vi "QModbus.vi"(9 "Main Process Class in":refnum<class "Main Class.lvclass">) -> ()   [LabVIEW 2019]
uses:
  Main Class.lvclass
  LLB/Commonly VI/Main Glb.vi
  LLB/Commonly VI.lvlib
  Ctrl/ModbusCmd.ctl
  <vilib>/NI/Modbus Library/API/Master/Modbus Master.lvclass
panel:
  out "error IO":errorcluster
  in  "Boolean":bool
  out "Main Process Class out":refnum<class "Main Class.lvclass">
  out "queue out":refnum<queue>
  out "register values":u16[](array[numeric])
  out "discrete inputs":bool[](array[boolean])
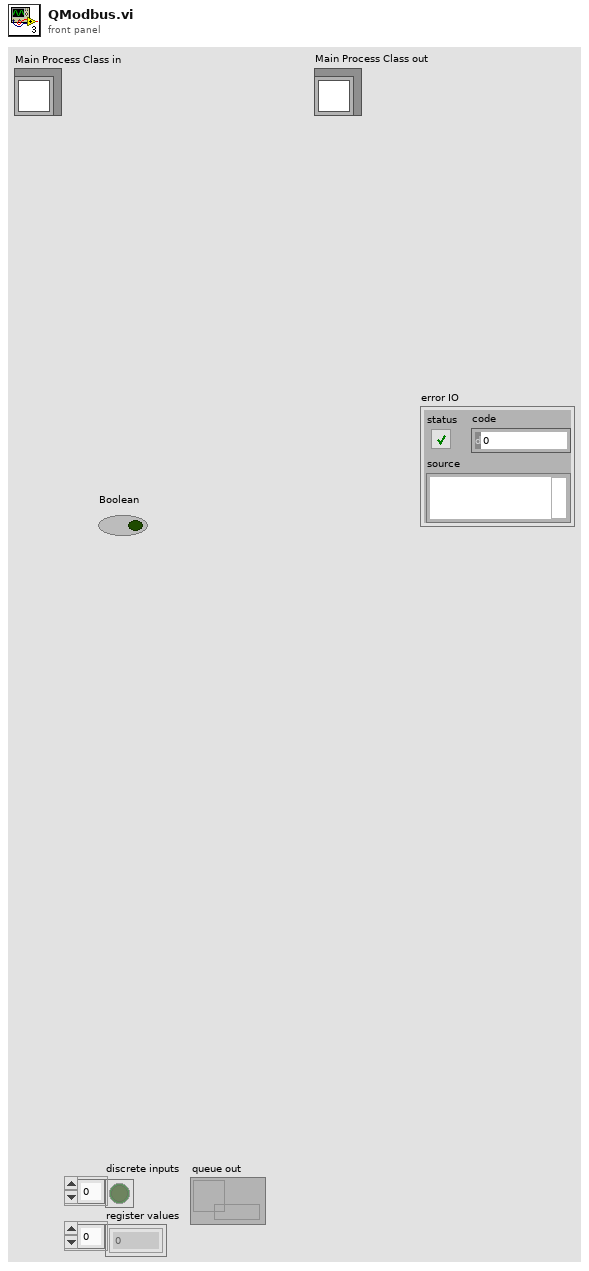
[diagram p1: front panel]
types:
  T1 = cluster{"AutoRunFlg":refnum<vi>, "Action Finish Flg":refnum<vi>, "Remaining Action":refnum<vi>, "Btn_AutoRun":refnum<vi>, "Manual Flg":refnum<vi>, "Sub Process Error":refnum<vi>}
  T2 = cluster{"starting address":u16, "coils to write":bool[]}
  T3 = typedef "ModbusCmd.ctl" = enum16{"Connect", "Disconnect", "Init", "Fetch Basic Objects", "Fetch Input Refisters", "Fetch Discrete Inputs", "Set Coils", "Set Holding Registers", "Write Single Holding", "Exit"}
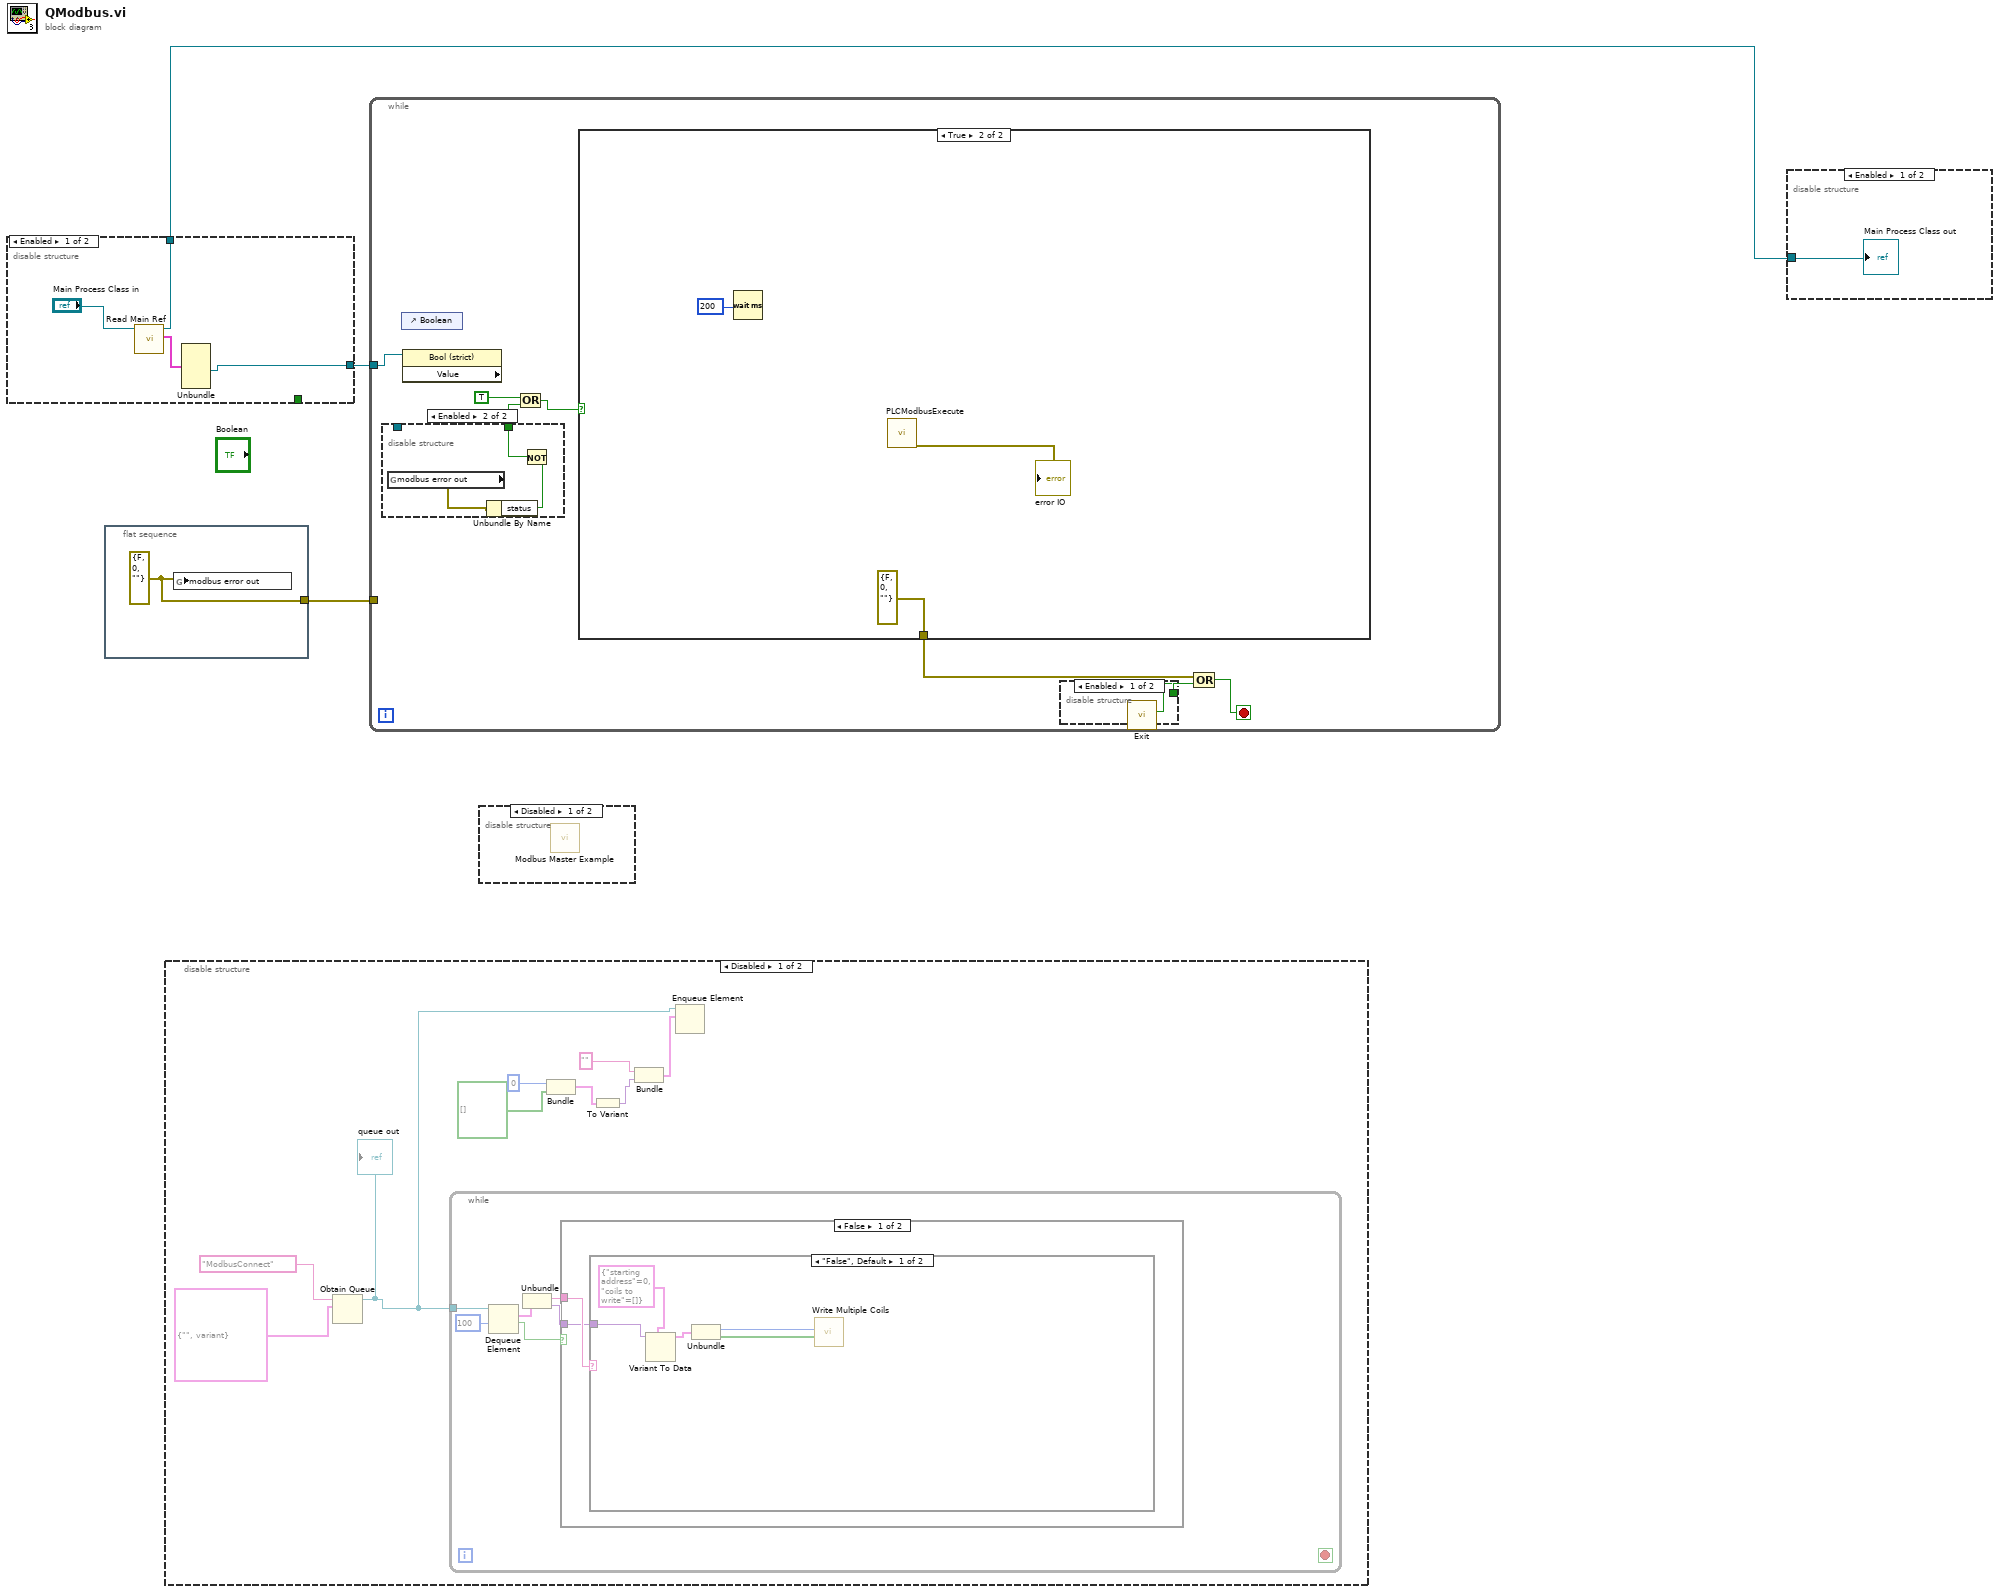
[diagram p0: block diagram]
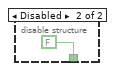
[diagram p4: hidden frame]
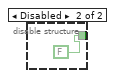
[diagram p5: hidden frame]
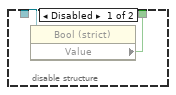
[diagram p6: hidden frame]
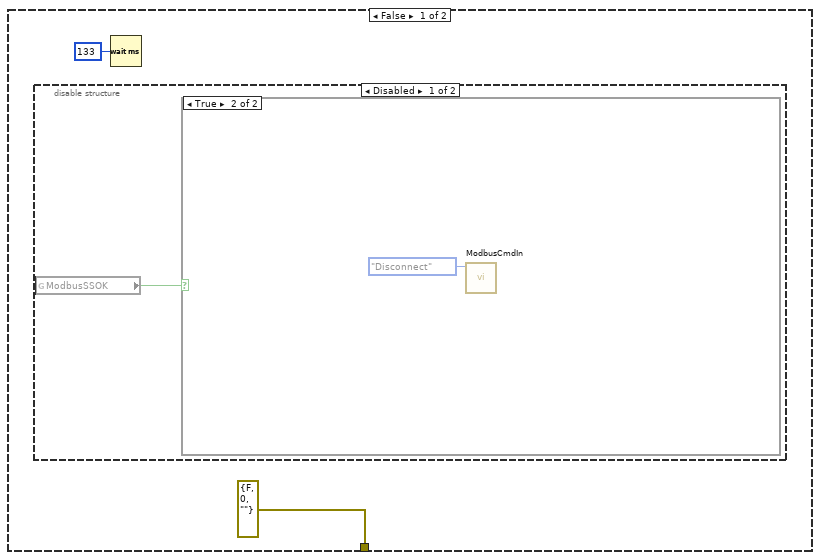
[diagram p7: hidden frame]
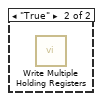
[diagram p10: hidden frame]
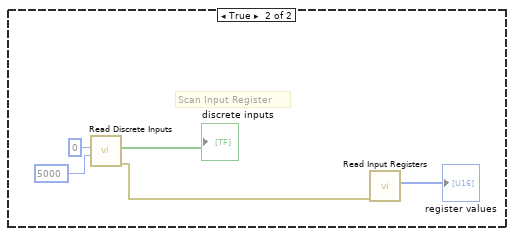
[diagram p11: hidden frame]
diagram:
  n1 = disable-structure shown="Enabled" {
    disable-tunnel: [w5 _] -> w3
    disable-tunnel: [_ FALSE] -> _
    disable-tunnel: [w4 _] -> w2
    frame Enabled {
      n2 = call-dynamic "Read Main Ref.vi"("Main Process Class in"="Main Process Class in") -> ("Main Ref"=w6:T1, "Main Process Class out"=w5:refnum<class "Main Class.lvclass">)  [unwired: 8 in, 1 out]
      n3 = Unbundle(w6) -> ("Btn_AutoRun"=w4:refnum<vi>)  [unwired: 5 out]
    }
    frame Disabled {
    }
  }
  n4 = flat-sequence {
    tunnel: [w9] -> w1
    frame #0 {
      w9 = errorcluster {"status"=FALSE, "code"=0, "source"=""} ("error out")
      n5 = global write "Main Glb.vi" "modbus error out"(w9) -> ()
    }
  }
  n6 = disable-structure shown="Disabled" {
    frame Disabled {
      n7 = Obtain Queue(name (unnamed)="ModbusConnect", element data type=cluster{string, variant} {"", variant}) -> (queue out=w10:refnum<queue>)  [unwired: 3 in, 2 out]
      "queue out" <- w10
      n8 = while {
        tunnel: w10 -> [w22]
        stop <- _ stop-if-true
        n9 = Dequeue Element(queue=w22, timeout in ms (-1)=100) -> (element=w21:cluster{string, variant}, timed out?=w23:bool)  [unwired: 1 in, 2 out]
        n10 = Unbundle(w21) -> (w20:string, w19:variant)
        n11 = case shown="False" w23 {
          tunnel: w20 -> [w26 _]
          tunnel: w19 -> [w25 _]
          frame False {
            n12 = case shown="\"False\", Default" w26 {
              tunnel: w25 -> [w31 _]
              frame "False", Default {
                n13 = Variant To Data(type=T2 {"starting address"=0, "coils to write"=[]} ("output cluster"), Variant=w31) -> (data=w29:T2)  [unwired: 1 in, 1 out]
                n14 = Unbundle(w29) -> ("starting address"=w28:u16, "coils to write"=w27:bool[])
                n15 = call-dynamic "Write Multiple Coils.vi"("coils to write"=w27, "starting address"=w28) -> ()  [unwired: 8 in, 2 out]
              }
              frame "True" {
                n16 = call-dynamic "Write Multiple Holding Registers.vi"() -> ()  [unwired: 10 in, 2 out]
              }
            }
          }
          frame True {
            # "Scan Input Register"
            n17 = call-dynamic "Read Discrete Inputs.vi"("number of inputs"=u16 5000 ("starting address"), "starting address"=u16 0) -> ("error out"=w33:errorcluster, "discrete inputs"=→"discrete inputs":bool[])  [unwired: 7 in, 1 out]
            n18 = call-dynamic "Read Input Registers.vi"("error in"=w33) -> ("register values"=→"register values":u16[])  [unwired: 8 in, 2 out]
          }
        }
      }
      n19 = Bundle("starting address"=u16 0, "coils to write"=bool[] []) -> (w15:T2)  [unwired: 1 in]
      n20 = To Variant(anything=w15) -> (Variant=w14:variant)
      n21 = Bundle("", "Variant"=w14) -> (w13:cluster{string, "Variant":variant})  [unwired: 1 in]
      n22 = Enqueue Element(queue=w10, element=w13) -> ()  [unwired: 2 in, 3 out]
    }
    frame Enabled {
    }
  }
  n23 = while {
    tunnel: w2 -> [w41]
    tunnel: w1 -> [_]
    stop <- w42 stop-if-true
    n24 = disable-structure shown="Enabled" {
      disable-tunnel: _ -> [w47 _]
      disable-tunnel: [w46 w48] -> w38
      frame Disabled {
        n25 = property class="Bool (strict)"(reference=w47) -> ("Value"=w46:bool)  [unwired: 1 in, 2 out]
      }
      frame Enabled {
        n26 = global read "Main Glb.vi" "modbus error out"() -> (w50:errorcluster)
        n27 = Unbundle By Name(w50) -> ("status"=w49:bool)
        n28 = Not(x=w49) -> (.not. x?=w48:bool)
      }
    }
    n29 = control-ref of="Boolean"() -> ()  [unwired: 1 out]
    n30 = property class="Bool (strict)" props=["Value"](reference=w41) -> ()  [unwired: 1 in, 3 out]
    n31 = Or(x=TRUE, y=w38) -> (x .or. y?=w37:bool)
    n32 = case shown="True" w37 {
      tunnel: [errorcluster {"status"=FALSE, "code"=0, "source"=""} ("error out") errorcluster {"status"=FALSE, "code"=0, "source"=""} ("error out")] -> w40
      frame False {
        n33 = disable-structure shown="Disabled" {
          frame Disabled {
            n34 = global read "Main Glb.vi" "ModbusSSOK"() -> (w53:bool)
            n35 = case shown="True" w53 {
              frame False {
              }
              frame True {
                n36 = call "ModbusCmdIn.vi"("Enum"=ModbusCmd."Disconnect") -> ()  [unwired: 10 in, 1 out]
              }
            }
          }
          frame Enabled {
          }
        }
        n37 = Wait (ms)(milliseconds to wait=u32 133) -> ()  [unwired: 1 out]
      }
      frame True {
        n38 = Wait (ms)(milliseconds to wait=200) -> ()  [unwired: 1 out]
        n39 = call "PLCModbusExecute.vi"() -> ("error IO"=→"error IO":errorcluster)  [unwired: 11 in]
      }
    }
    n40 = disable-structure shown="Enabled" {
      disable-tunnel: [w44 FALSE] -> w43
      frame Enabled {
        n41 = call "Exit.vi"() -> ("ExitOut"=w44:bool)  [unwired: 11 in]
      }
      frame Disabled {
      }
    }
    n42 = Compound Arithmetic op=OR(w40, w43) -> (w42:bool)
  }
  n43 = disable-structure shown="Disabled" {
    frame Disabled {
      n44 = call <vilib>:"Modbus Master Example.vi"() -> ()  [unwired: 12 in]
    }
    frame Enabled {
    }
  }
  n45 = disable-structure shown="Enabled" {
    disable-tunnel: w3 -> [w58 _]
    frame Enabled {
      "Main Process Class out" <- w58
    }
    frame Disabled {
    }
  }
